vi "CMN_toGRTD.vi"(2 "responseQ":string, 4 "Elements":u16[](array[numeric]), 5 "ms timeout (-1)":i32=-1, 7 "error in (no error)":errorcluster, 8 "Elements Read":u32, 9 "location":u64, 10 "argument":string, 11 "Command":string) -> (0 "error out":errorcluster)   [LabVIEW 2016]
panel:
  out "response":errorcluster
  in  "RTD struct":T1
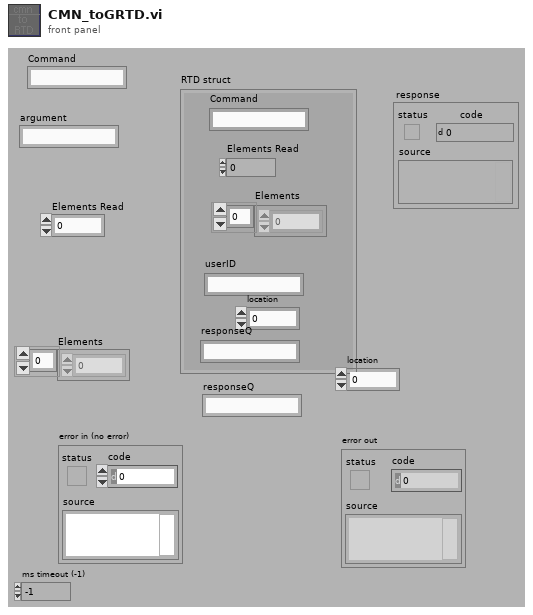
[diagram p1: front panel]
types:
  T1 = cluster{"Command":string, "Elements Read":u32, "Elements":u16[], "userID":string, "location":u64, "responseQ":string}
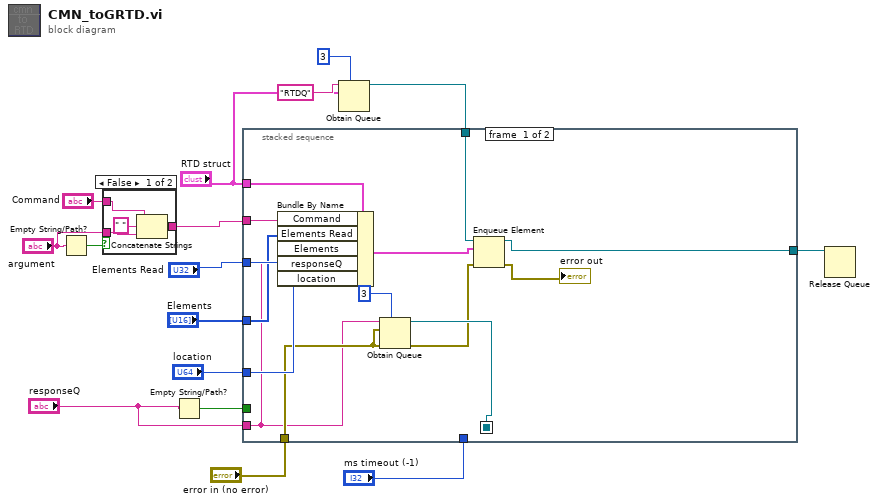
[diagram p0: block diagram]
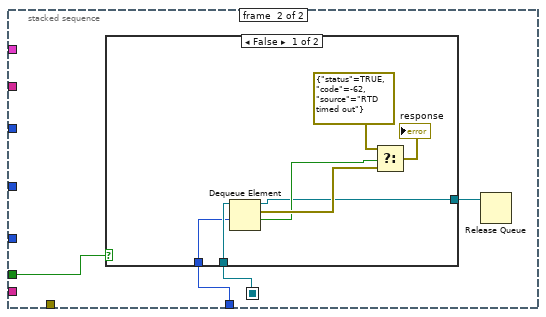
[diagram p3: hidden frame]
diagram:
  n1 = Empty String/Path?(string/path="argument") -> (empty?=w13:bool)
  n2 = case shown="False" w13 {
    tunnel: "Command" -> [w19 w21]
    tunnel: "argument" -> [w18 _]
    tunnel: [w17 w21] -> w10
    frame False {
      n3 = Concatenate Strings(w19, " ", w18) -> (w17:string)
    }
    frame True {
    }
  }
  n4 = Empty String/Path?(string/path="responseQ") -> (empty?=w7:bool)
  n5 = Obtain Queue(max queue size (-1, unlimited)=3, name (unnamed)="RTDQ", element data type="RTD struct") -> (queue out=w3:refnum<queue>)  [unwired: 2 in, 2 out]
  n6 = stacked-sequence {
    seq-local: [w29 _] -> [_ w36]
    tunnel: w10 -> [w35 _]
    tunnel: "Elements Read" -> [w34 _]
    tunnel: "Elements" -> [w33 _]
    tunnel: "RTD struct" -> [w32 _]
    tunnel: "location" -> [w31 _]
    tunnel: "ms timeout (-1)" -> [_ w37]
    tunnel: "error in (no error)" -> [w30 _]
    tunnel: w7 -> [_ w39]
    tunnel: "responseQ" -> [w28 _]
    tunnel: w3 -> [w27 _]
    tunnel: [w23 _] -> w2
    frame #0 {
      n7 = Bundle By Name(cluster=w32, "Command"=w35, "Elements Read"=w34, "Elements"=w33, "responseQ"=w28, "location"=w31) -> (w26:T1)
      n8 = Obtain Queue(max queue size (-1, unlimited)=3, name (unnamed)=w28, element data type=w30, error in (no error)=w30) -> (queue out=w29:refnum<queue>, error out=w24:errorcluster)  [unwired: 1 in, 1 out]
      n9 = Enqueue Element(queue=w27, element=w26, error in (no error)=w24) -> (queue out=w23:refnum<queue>, error out=→"error out":errorcluster)  [unwired: 2 out]
    }
    frame #1 {
      n10 = case shown="False" w39 {
        tunnel: w37 -> [w42 _]
        tunnel: w36 -> [w44 w47]
        tunnel: [w40 w47] -> w38
        frame False {
          n11 = Dequeue Element(queue=w44, timeout in ms (-1)=w42) -> (queue out=w40:refnum<queue>, element=w43:errorcluster, timed out?=w41:bool)  [unwired: 1 in, 1 out]
          n12 = Select(t=errorcluster {"status"=TRUE, "code"=-62, "source"="RTD timed out"}, s=w41, f=w43) -> (s? t:f=→"response":errorcluster)
        }
        frame True {
        }
      }
      n13 = Release Queue(queue=w38) -> ()  [unwired: 1 in, 4 out]
    }
  }
  n14 = Release Queue(queue=w2) -> ()  [unwired: 1 in, 4 out]
